vi "Timestamp for data.vi"() -> (1 "date/time string":string)   [LabVIEW 2015]
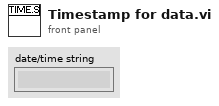
[diagram p1: front panel]
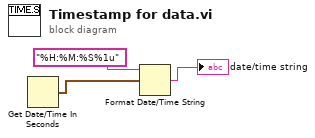
[diagram p0: block diagram]
diagram:
  n1 = Get Date/Time In Seconds() -> (seconds since 1Jan1904=w1:timestamp)
  n2 = Format Date/Time String(time format string (%c)="%H:%M:%S%1u", seconds (now)=w1) -> (date/time string=→"date/time string":string)  [unwired: 1 in]
